vi "Error Query.vi"(0 "VISA resource name":refnum<visa-resource-name>, 11 "error in (no error)":errorcluster) -> (4 "VISA resource name out":refnum<visa-resource-name>, 8 "Error":i32, 10 "Error Message":string, 15 "error out":errorcluster)   [LabVIEW 2010, in "Stanford Research PS300 Series.lvlib"]
doc: "This instrument does not support an error query and will return a warning if this VI is called."
uses:
  <instrlib>/Stanford Research PS300 Series/Stanford Research PS300 Series.lvlib
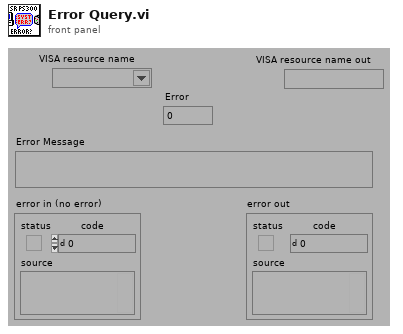
[diagram p1: front panel]
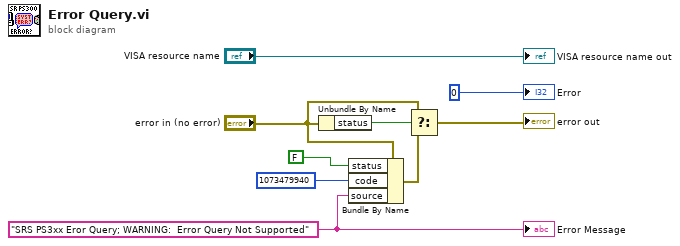
[diagram p0: block diagram]
diagram:
  w1 = "SRS PS3xx Eror Query; WARNING:  Error Query Not Supported" ("source")
  n1 = Unbundle By Name("error in (no error)") -> ("status"=w4:bool)
  n2 = Bundle By Name(cluster="error in (no error)", "status"=FALSE, "code"=1073479940, "source"=w1) -> (w5:errorcluster)
  n3 = Select(t="error in (no error)", s=w4, f=w5) -> (s? t:f=→"error out":errorcluster)
  "Error Message" <- w1
  "Error" <- 0
  "VISA resource name out" <- "VISA resource name"
